vi "SynapseAPI-Get Parameter Value (1D).vi"(0 "URL":string="http://localhost:24414", 5 "Gizmo":string, 7 "Parameter":string, 11 "error in (no error)":errorcluster) -> (8 "value":dbl[](array[numeric]), 15 "error out":errorcluster)   [LabVIEW 2015]
uses:
  <vilib>/httpClient/LabVIEWHTTPClient.lvlib
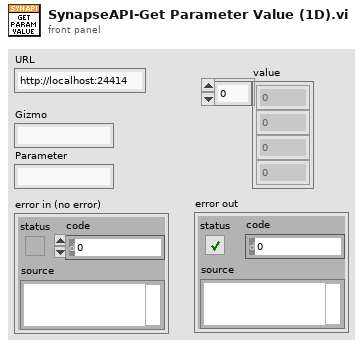
[diagram p1: front panel]
types:
  T1 = typedef "LabVIEWHTTPClient.lvlib/ClientHandle.ctl" = refnum<k1>
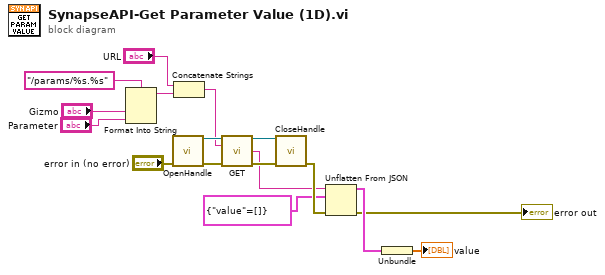
[diagram p0: block diagram]
diagram:
  n1 = Format Into String(format string="/params/%s.%s", "Gizmo", "Parameter") -> (resulting string=w6:string)  [unwired: 2 in, 1 out]
  n2 = call <vilib>:"OpenHandle.vi"("error in (no error)"="error in (no error)") -> ("client handle out"=w15:T1, "error out"=w14:errorcluster)  [unwired: 13 in]
  n3 = Concatenate Strings("URL", w6) -> (w8:string)
  n4 = call <vilib>:"GET.vi"("client handle"=w15, "url"=w8, "error in (no error)"=w14) -> ("client handle out"=w16:T1, "body"=w11:string, "error out"=w17:errorcluster)  [unwired: 9 in, 1 out]
  n5 = call <vilib>:"CloseHandle.vi"("client handle"=w16, "error in (no error)"=w17) -> ("error out"=w13:errorcluster)  [unwired: 13 in]
  n6 = Unflatten From JSON(JSON string=w11, type and defaults=cluster{"value":dbl[]} {"value"=[]} ("Cluster"), error in (no error)=w13) -> (value=w9:cluster{"value":dbl[]}, error out=→"error out":errorcluster)  [unwired: 4 in]
  n7 = Unbundle(w9) -> ("value"=→"value":dbl[])
